vi "Write Default Value.vi"(8 "error in":errorcluster, 10 "default value":dbl, 11 "PWM channel in":refnum<class "PWM Channel.lvclass">) -> (0 "error out":errorcluster, 3 "PWM channel out":refnum<class "PWM Channel.lvclass">)   [LabVIEW 2017, in "Scan Engine Scripting.lvlib" / "PWM Channel.lvclass"]
doc: "Writes the default value for the channel in its private data."
uses:
  PWM Channel.lvclass
  PWM Channel.lvclass/PWM Channel.ctl
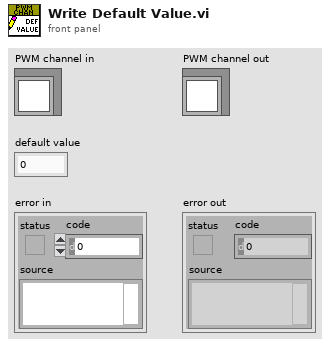
[diagram p1: front panel]
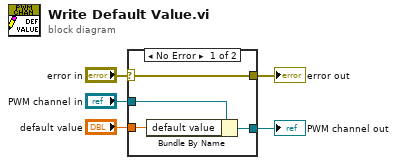
[diagram p0: block diagram]
diagram:
  n1 = case shown="No Error" "error in" {
    selector: "error in" -> [w9 w10]
    tunnel: [w9 w10] -> w4
    tunnel: [w7 w11] -> w2
    tunnel: "PWM channel in" -> [w8 w11]
    tunnel: "default value" -> [w6 _]
    frame No Error {
      n2 = Bundle By Name(cluster=w8, "default value"=w6) -> (w7:refnum<class "PWM Channel.lvclass">)
    }
    frame Error {
    }
  }
  "error out" <- w4
  "PWM channel out" <- w2
